vi "Mono Init.vi"(8 "error in (no error)":errorcluster, 11 "Mono In":refnum<class "Monochromator.lvclass">) -> (0 "error out":errorcluster, 2 "new is initialized?":bool, 3 "mono is initialized?":bool)   [LabVIEW 2020, in "Examples.lvlib"]
doc: "\"Mono init\" tells the mono to start the homing procedure. This calls completes immediately but only kicks off the homing procedure. It is necessary to query the mono afterwards to check when the homing has completed."
uses:
  Examples.lvlib
  1e589c04-ee94-437c-90d0-11a3ef27d9f2.vi
  Classes/Mono/Monochromator.lvclass
  98d9e02b-2768-4993-9cff-527122a95b91.vi
panel:
  in  "Stop":bool
  # "Connector Pane"
  # "Locals"
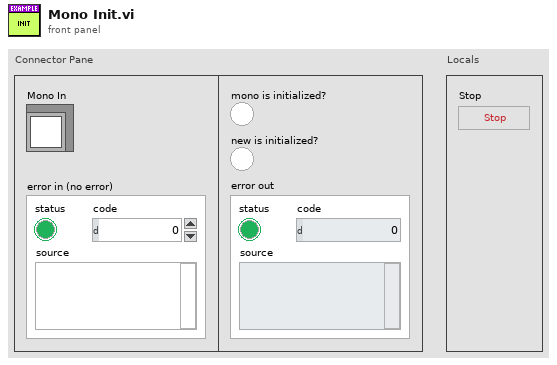
[diagram p1: front panel]
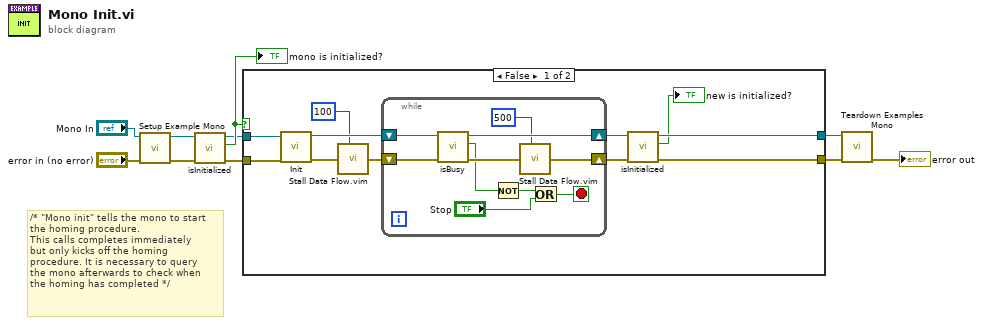
[diagram p0: block diagram]
diagram:
  # "/* \"Mono init\" tells the mono to start\nthe homing procedure.\nThis calls completes immediately\nbut only kicks off the homing\nprocedure. It is necessary to query \nthe mono afterwards to check when \nthe homing has completed */"
  n1 = call "Setup Example Mono.vi"("error in (no error)"="error in (no error)", "Mono In"="Mono In") -> ("error out"=w4:errorcluster, "Mono Out"=w5:refnum<class "Monochromator.lvclass">)  [unwired: 6 in, 2 out]
  n2 = call "isInitialized.vi"("error in (no error)"=w4, "Monochromator in"=w5) -> ("error out"=w2:errorcluster, "mono is initialized?"=w3:bool, "Monochromator out"=w1:refnum<class "Monochromator.lvclass">)  [unwired: 7 in]
  "mono is initialized?" <- w3
  n3 = case shown="False" w3 {
    tunnel: [w19 w33] -> w7
    tunnel: [w18 w32] -> w6
    tunnel: w2 -> [w12 w33]
    tunnel: w1 -> [w11 w32]
    frame False {
      n4 = call "Init.vi"("error in (no error)"=w12, "Monochromator in"=w11) -> ("error out"=w21:errorcluster, "Monochromator out"=w20:refnum<class "Monochromator.lvclass">)  [unwired: 6 in, 2 out]
      n5 = call "Stall Data Flow.vim"("value in"=w21, "milliseconds to wait"=u32 100) -> ("value out"=w16:errorcluster)  [unwired: 1 out]
      n6 = while {
        shift-right: [w27] -> w14
        shift-left: w16 -> [w29]
        shift-right: [w30] -> w15
        shift-left: w20 -> [w28]
        stop <- w24 stop-if-true
        n7 = call "isBusy.vi"("error in (no error)"=w29, "Monochromator in"=w28) -> ("error out"=w31:errorcluster, "mono is busy?"=w25:bool, "Monochromator out"=w30:refnum<class "Monochromator.lvclass">)  [unwired: 7 in]
        n8 = Not(x=w25) -> (.not. x?=w22:bool)
        n9 = call "Stall Data Flow.vim"("value in"=w31, "milliseconds to wait"=u32 500) -> ("value out"=w27:errorcluster)  [unwired: 1 out]
        n10 = Or(x=w22, y="Stop") -> (x .or. y?=w24:bool)
      }
      n11 = call "isInitialized.vi"("error in (no error)"=w14, "Monochromator in"=w15) -> ("error out"=w19:errorcluster, "mono is initialized?"=→"new is initialized?":bool, "Monochromator out"=w18:refnum<class "Monochromator.lvclass">)  [unwired: 7 in]
    }
    frame True {
    }
  }
  n12 = call "Teardown Examples Mono.vi"("error in (no error)"=w7, "Monochromator in"=w6) -> ("error out"=→"error out":errorcluster)  [unwired: 9 in]
